vi "Programming Relays.vi"(8 "error in (no error)":errorcluster, 10 "Connect (False)":bool=TRUE, 11 "Application in":refnum<class "Application.lvclass">) -> (0 "error out":errorcluster)   [LabVIEW 2015, in "LCM Single-Up MTS Programming.lvclass"]
uses:
  LCM Single-Up MTS Programming.lvclass
  Classes/Application/Class/Application.lvclass
  CBTF Applications/SmartCast Testing/Main/LCM Single-Up/Application/Application/Class/typedefs/Instrument Selector -- Enum.ctl
  Classes/Instruments/Relay Control/Class/Relay Control.lvclass
  CBTF Applications/SmartCast Testing/Main/LCM Single-Up/Application/Application/Class/LCM Single-Up.lvclass
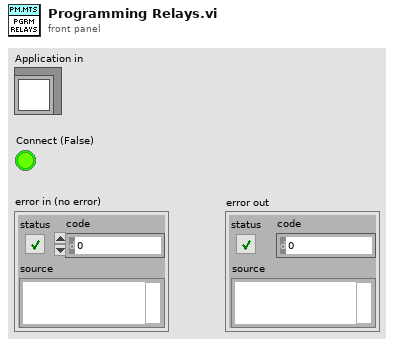
[diagram p1: front panel]
types:
  T1 = typedef "LCM Single-Up.lvlib/LCM Single-Up.lvclass/Instrument Selector -- Enum.ctl" = enum16{"Relay", "MIO Device", "I2C Device", "Thermocouple"}
  T2 = typedef "Application.lvlib/App Properties.lvclass/Class Properties -- Cluster.ctl" = cluster{"UUT Info":T3[], "Test Information":refnum<vi>, "Test Complete Event":refnum<user-event>, "Shop Floor System":refnum<class "Shop Floor System.lvclass">, "Gold Board":refnum<class "Golden Board.lvclass">, "Test Recipe":refnum<class "Test Recipe.lvclass">, "Instruments":refnum<class "Base Class.lvclass">[], "Mode":T4, "Test Results":cluster{"Pass":bool[], "Fail Codes":string[]}, "Station Config":refnum<class "Station Config.lvclass">}
  T3 = typedef "Application.lvlib/App Properties.lvclass/UUT Reference -- Cluster.ctl" = cluster{"Serial Number Reference":refnum<vi>, "Status Message Reference":refnum<vi>}
  T4 = typedef "Application.lvlib/Application.lvclass/Op Mode -- Enum.ctl" = u16
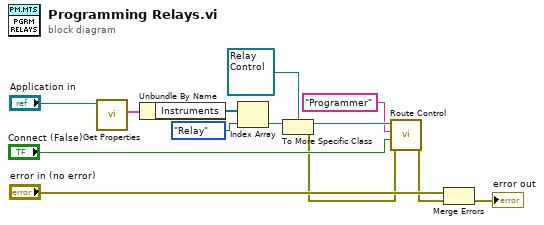
[diagram p0: block diagram]
diagram:
  n1 = call "Get Properties.vi"("Acrobat Template in"="Application in") -> ("Class Properties"=w11:T2)  [unwired: 8 in, 2 out]
  n2 = Unbundle By Name(w11) -> ("Instruments"=w9:refnum<class "Base Class.lvclass">[])
  n3 = Index Array(array=w9, index=Instrument_Selector_--_Enum."Relay" ("Instrument")) -> (element=w10:refnum<class "Base Class.lvclass">)
  n4 = To More Specific Class(target class=refnum<class "Relay Control.lvclass"> refnum ("Relay Control.lvlib:Relay Control.lvclass"), reference=w10) -> (specific class reference=w5:refnum<class "Relay Control.lvclass">, error out=w2:errorcluster)  [unwired: 1 in]
  n5 = call "Route Control.vi"("error in (no error)"=w2, "Connect (False)"="Connect (False)", "Route Name"="Programmer", "Relay Control in"=w5) -> ("error out"=w1:errorcluster)  [unwired: 6 in, 1 out]
  n6 = Merge Errors("error in (no error)", w1) -> (→"error out":errorcluster)
